vi "Global VI.vi"() -> ()   [LabVIEW 2013]
panel:
  out "Users":string[][](array[string])=[["Operator", "Maint", "Admin"], ["Password", "123Abc!", "Admin"], ["1", "2", "2"]]
  out "Faulted Status":bool
  in  "Robot Status String":string="System Idle"
  in  "Access Level":u16(ring) items=["No Access", "Operator", "Engineer/Tech"]
  out "Operator":string="Admin"
  out "Screen Width":i16=1280
  in  "# of Screens":i16=2
  out "SubVIs":string[](array[string])=["Alarms_u_1.vi", "Home_u_0.vi", "Maint_u_2.vi"]
  in  "Monitor":u16
  in  "stop":bool
  out "Page Names":string[](array[string])=["Alarms", "Home", "Maint"]
  in  "Page":i16=2
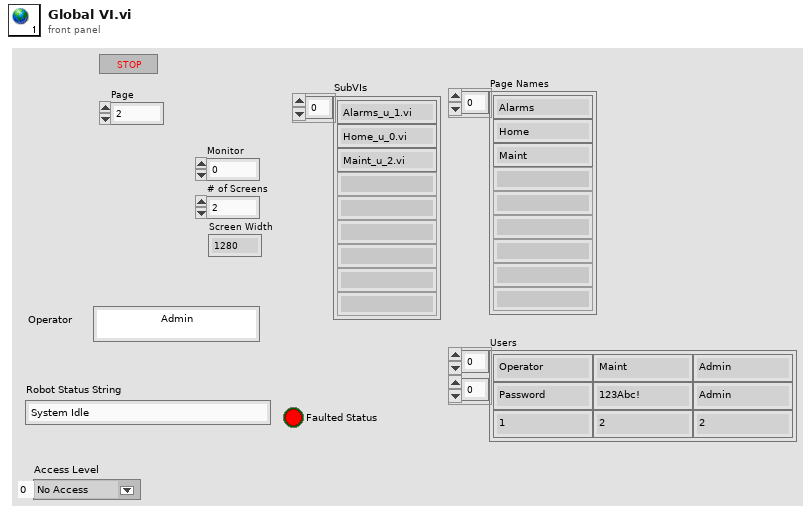
[diagram p1: front panel]
diagram:
